vi "Loop.vi"() -> ()   [LabVIEW 2018]
panel:
  out "Value History":dbl(graph)
  in  "stop":bool
  in  "millisecond delay":dbl(slide) scale=10.0..300.0
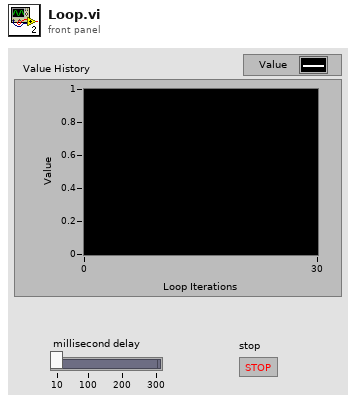
[diagram p1: front panel]
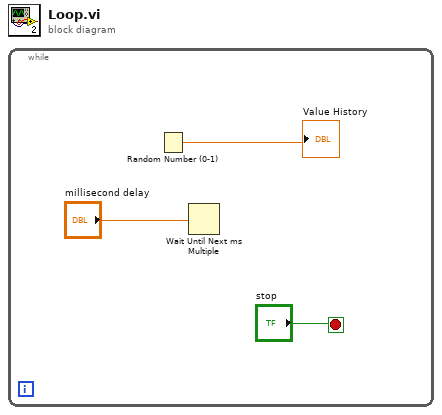
[diagram p0: block diagram]
diagram:
  n1 = while {
    stop <- "stop" stop-if-true
    n2 = Random Number (0-1)() -> (number: 0 to 1=→"Value History":dbl)
    n3 = Wait Until Next ms Multiple(millisecond multiple="millisecond delay") -> ()  [unwired: 1 out]
  }
